vi "DSF.Memory.Buffer.Errors.Invalid Buffer.vi"(7 "calling vi name":string, 8 "error in (no error)":errorcluster, 11 "Buffer in":refnum<class "DSF.Memory.Buffer.lvclass">) -> (0 "error out":errorcluster, 3 "Buffer out":refnum<class "DSF.Memory.Buffer.lvclass">)   [LabVIEW 2016, in "DSF.Memory.lvlib" / "DSF.Memory.Buffer.lvclass"]
uses:
  DSF.Memory.Buffer.lvclass
  Submodules/Memory Manager/Source/Submodules/SEH/Source/VIs/Static Error Handling.Error Cluster Constant (512B).vi
  Constants/DSF.Common.Constants.Library Name.vi
  Submodules/Memory Manager/Source/Submodules/SEH/Source/Static Error Handling.lvlib
  DSF.Common.lvlib
  Submodules/Memory Manager/Source/Submodules/SEH/Source/VIs/Static Error Handling.Source Buffer.Write.Numeric.Scalar.Base10 (I8).vi
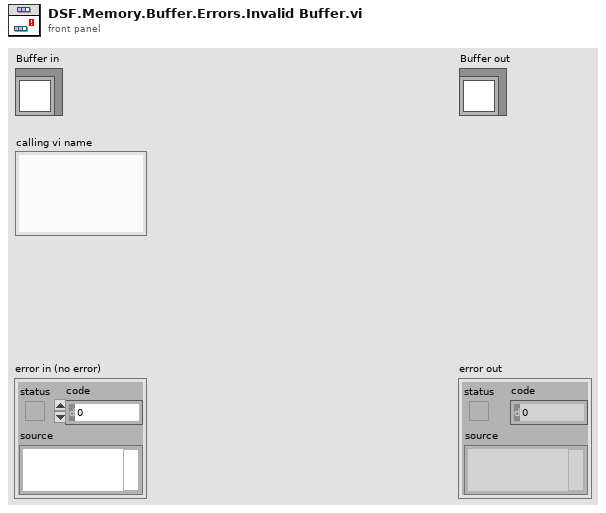
[diagram p1: front panel]
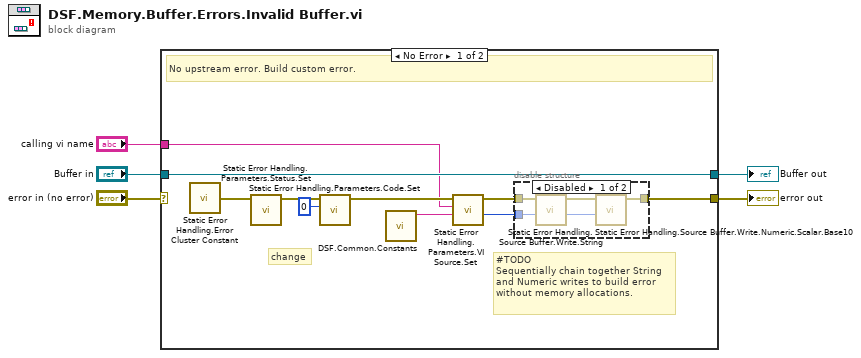
[diagram p0: block diagram]
diagram:
  n1 = case shown="No Error" "error in (no error)" {
    selector: "error in (no error)" -> [_ w22]
    tunnel: "Buffer in" -> [w14 w23]
    tunnel: [w14 w23] -> w4
    tunnel: [w7 w22] -> w3
    tunnel: "calling vi name" -> [w9 _]
    frame No Error {
      # "#TODO\nSequentially chain together String and Numeric writes to build error without memory allocations."
      # "change"
      # "No upstream error. Build custom error."
      n2 = call-poly "Static Error Handling.Error Cluster Constant.vi"() -> ("error out"=w15:errorcluster)  [unwired: 1 in]
      n3 = call "Static Error Handling.Parameters.Status.Set.vi"("error in"=w15) -> ("error out"=w11:errorcluster)  [unwired: 10 in]
      n4 = call "Static Error Handling.Parameters.Code.Set.vi"("code"=0, "error in"=w11) -> ("error out"=w10:errorcluster)  [unwired: 9 in]
      n5 = call-poly "DSF.Common.Constants.vi"() -> ("Library Name"=w13:string)  [unwired: 11 in]
      n6 = call "Static Error Handling.Parameters.VI Source.Set.vi"("library name (\"\")"=w13, "vi name"=w9, "error in"=w10) -> ("new offset"=w6:i32, "error out"=w8:errorcluster)  [unwired: 7 in]
      n7 = disable-structure shown="Disabled" {
        disable-tunnel: w8 -> [w20 w21]
        disable-tunnel: [w18 w21] -> w7
        disable-tunnel: w6 -> [w17 _]
        frame Disabled {
          n8 = call "Static Error Handling.Source Buffer.Write.String.vi"("offset"=w17, "error in"=w20) -> ("new offset"=w16:i32, "error out"=w19:errorcluster)  [unwired: 8 in]
          n9 = call-poly "Static Error Handling.Source Buffer.Write.Numeric.Scalar.Base10.vi"("offset"=w16, "error in"=w19) -> ("error out"=w18:errorcluster)  [unwired: 8 in, 1 out]
        }
        frame Enabled {
        }
      }
    }
    frame Error {
      # "Upstream error. Pass through."
    }
  }
  "error out" <- w3
  "Buffer out" <- w4
